vi "ColorDetectionGlobalVariable.vi"() -> ()   [LabVIEW 2016]
panel:
  in  "Black Status":dbl
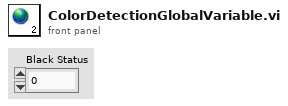
[diagram p1: front panel]
diagram:
